vi "Get Connections - 1Pin 1Conn.vi"(8 "error in":errorcluster, 9 "site":i32=-1, 10 "pin or relay name":string, 11 "session reservation in":refnum<class "Session Reservation.lvclass">) -> (0 "error out":errorcluster, 2 "connection":T1, 3 "session reservation out":refnum<class "Session Reservation.lvclass">)   [LabVIEW 2020, in "Keysight 34401A DMM Instrument.lvlib"]
doc: "Gets the 34401 connection information for the given <b>pin or relay name</b> and <b>site</b>. If the <b>pin or relay name</b> input is unwired, the connection information for all pins on the given <b>site</b> will be returned. If the <b>site</b> input is unwired, the connection information for the given <b>pin or relay name</b> for all sites will be returned. If both the <b>pin or relay name</b> and <b>site</b> inputs are unwired, the connection information for all pins and on all sites will be returned.\n\nIf you have not called <b>Create Sessions.vi</b> prior to calling this VI, the connection information will be returned with the correct information but will have an invalid session.\n\nThis VI returns an error if multiple connections match the inputs. Use <b>Get Connections - 1Pin MConn.vi</b> to get multiple connections from a single pin."
uses:
  Keysight 34401A DMM Instrument.lvlib
  <vilib>/MeasurementLink/MeasurementLink Session Management/Session Reservation/Session Reservation.lvclass
  Connection with Session.ctl
  <vilib>/MeasurementLink/MeasurementLink Session Management/Session Reservation/Connection.ctl
  Instrument/Instrument.lvclass
  C:/Program Files/National Instruments/LabVIEW 2020/vi.lib/MeasurementLink/MeasurementLink Instrument/IInstrument/IInstrument.lvclass
  86b200b6-28cb-4bb1-b3a2-edbec9fb38cc.vi
  86b200b6-28cb-4bb1-b3a2-edbec9fb38cc.vi/d089b476-b30c-4b91-b2ff-fbae0086b065.vi
  <vilib>/MeasurementLink/MeasurementLink Session Management/Session Reservation/Pin to Pin Array.vi
  <vilib>/MeasurementLink/MeasurementLink Session Management/Session Reservation/Get Connections Dispatcher.vi
  <vilib>/MeasurementLink/MeasurementLink Measurement Server/Helpers/Error Strings Global Internal.vi
  <vilib>/Utility/error.llb/Error Cluster From Error Code.vi
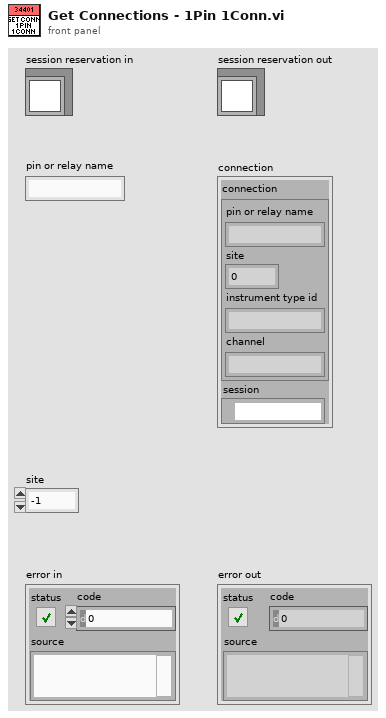
[diagram p1: front panel]
types:
  T1 = typedef "Keysight 34401A DMM Instrument.lvlib/Connection with Session.ctl" = cluster{"connection":T2, "session":refnum<visa-resource-name>}
  T2 = typedef "MeasurementLink Session Management.lvlib/Session Reservation.lvclass/Connection.ctl" = cluster{"pin or relay name":string, "site":i32, "instrument type id":string, "channel":string}
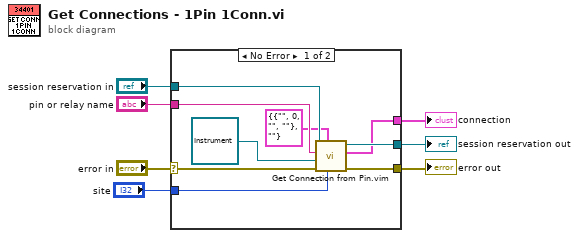
[diagram p0: block diagram]
diagram:
  n1 = case shown="No Error" "error in" {
    selector: "error in" -> [w10 w17]
    tunnel: "session reservation in" -> [w13 w18]
    tunnel: "pin or relay name" -> [w11 _]
    tunnel: [w14 w17] -> w4
    tunnel: [w16 w18] -> w3
    tunnel: [w15 _] -> w1
    tunnel: "site" -> [w12 _]
    frame No Error {
      n2 = call "Get Connection from Pin.vim"("site"=w12, "connection type"=T1 {"connection"={"pin or relay name"="", "site"=0, "instrument type id"="", "channel"=""}, "session"=""} ("connection with session"), "error in"=w10, "instrument"=refnum<class "Instrument.lvclass"> refnum ("MeasurementLink 34401.lvlib:Instrument.lvclass"), "pin or relay name"=w11, "session reservation in"=w13) -> ("error out"=w14:errorcluster, "connection"=w15:T1, "session reservation out"=w16:refnum<class "Session Reservation.lvclass">)  [unwired: 3 in]
    }
    frame Error {
    }
  }
  "error out" <- w4
  "session reservation out" <- w3
  "connection" <- w1
